vi "Send TCP Param.vi"(8 "error in (no error)":errorcluster, 11 "Server in":refnum<class "Server.lvclass">) -> (0 "error out":errorcluster, 3 "Server out":refnum<class "Server.lvclass">)   [LabVIEW 2018, in "Server.lvclass"]
uses:
  Server.lvclass
  Server.lvclass/Server.ctl
panel:
  in  "Cluster":cluster{"Address":string, "Remote Port":u32}
  out "output cluster":cluster{"Address":string, "Remote Port":u32}
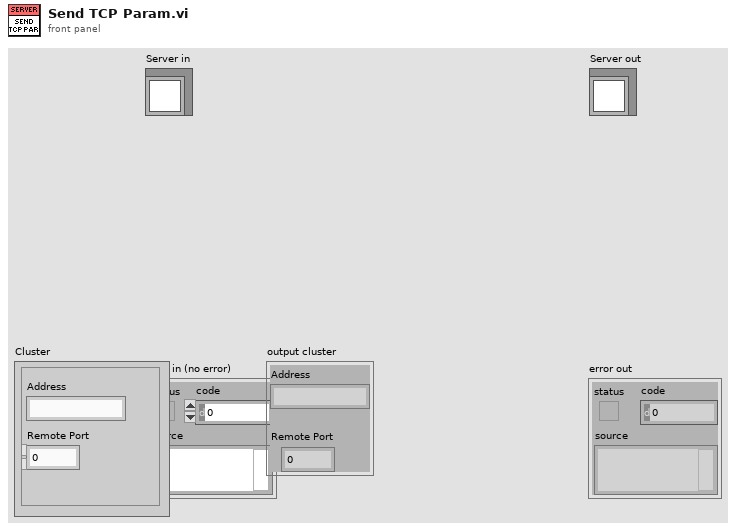
[diagram p1: front panel]
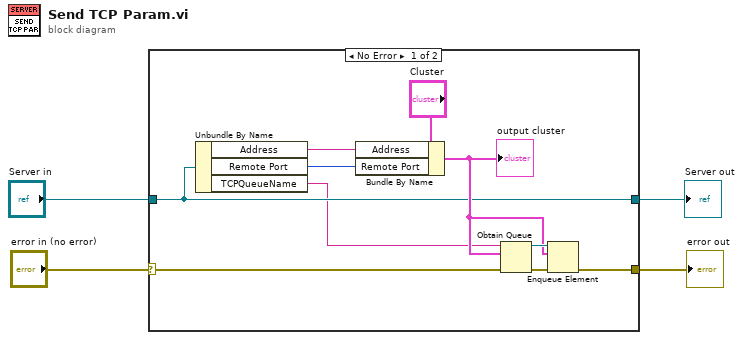
[diagram p0: block diagram]
diagram:
  n1 = case shown="No Error" "error in (no error)" {
    selector: "error in (no error)" -> [w8 w16]
    tunnel: [w10 w16] -> w1
    tunnel: [w9 w15] -> w2
    tunnel: "Server in" -> [w9 w15]
    frame No Error {
      n2 = Unbundle By Name(w9) -> ("Address"=w7:string, "Remote Port"=w6:u32, "TCPQueueName"=w5:string)
      n3 = Bundle By Name(cluster="Cluster", "Address"=w7, "Remote Port"=w6) -> (w11:cluster{"Address":string, "Remote Port":u32})
      "output cluster" <- w11
      n4 = Obtain Queue(name (unnamed)=w5, element data type=w11, error in (no error)=w8) -> (queue out=w14:refnum<queue>, error out=w13:errorcluster)  [unwired: 2 in, 1 out]
      n5 = Enqueue Element(queue=w14, element=w11, error in (no error)=w13) -> (error out=w10:errorcluster)  [unwired: 1 in, 2 out]
    }
    frame Error {
    }
  }
  "error out" <- w1
  "Server out" <- w2
